vi "RANGE Accuracy At Zero.vi"(9 "Accuracy Full Scale":dbl, 10 "Accuracy Reading":dbl, 11 "Meter Size":dbl) -> (3 "SLPMErrZero":dbl)   [LabVIEW 2016]
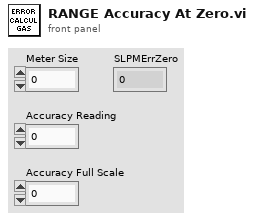
[diagram p1: front panel]
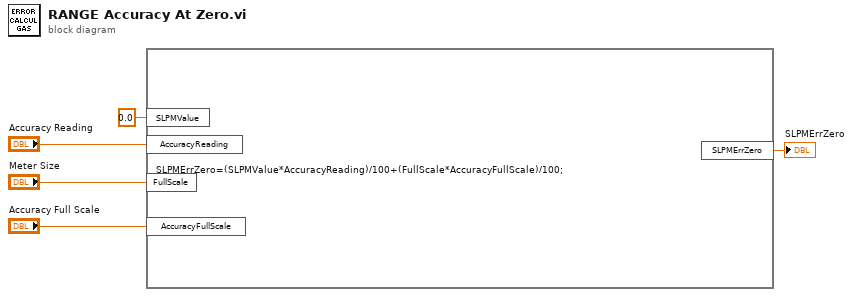
[diagram p0: block diagram]
diagram:
  n1 = formula code="SLPMErrZero=(SLPMValue*AccuracyReading)/100+(FullScale*AccuracyFullScale)/100;"("SLPMValue"=0.0 ("input variable"), "AccuracyReading"="Accuracy Reading", "FullScale"="Meter Size", "AccuracyFullScale"="Accuracy Full Scale") -> ("SLPMErrZero"=→"SLPMErrZero":dbl)
